vi "Snap.vi"(8 "error in (no error)":errorcluster, 11 "VisionUI in":refnum<class "VisionUI.lvclass">) -> (0 "error out":errorcluster, 3 "VisionUI out":refnum<class "VisionUI.lvclass">)   [LabVIEW 2021, in "VisionUI.lvlib" / "VisionUI.lvclass"]
uses:
  VisionUI.lvclass
  C:/Users/alan0/Desktop/WebSocket/Actors/Vision/Vision/Vision.lvclass
  VisionUI.lvclass/VisionUI.ctl
  Vision/Vision/Vision.lvclass
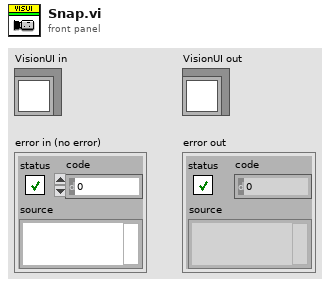
[diagram p1: front panel]
types:
  T1 = typedef "IMAQ Image.ctl" = refnum<image>
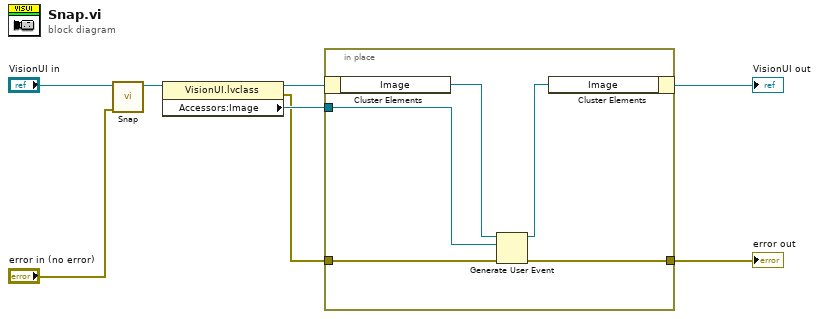
[diagram p0: block diagram]
diagram:
  n1 = call-parent "Snap.vi"("error in (no error)"="error in (no error)", "Vision in"="VisionUI in") -> ("Vision out"=w8:refnum<class "VisionUI.lvclass">)  [unwired: 8 in, 1 out]
  n2 = property class="VisionUI.lvclass"(reference=w8) -> (reference out=w5:refnum<class "VisionUI.lvclass">, error out=w2:errorcluster, "Accessors:Image"=w3:T1)  [unwired: 1 in]
  n3 = in-place {
    in-place-border: w3 -> [w11]
    in-place-border: w2 -> [w10]
    in-place-border: [w9] -> w1
    n4 = in-place-cluster #1(w5) -> ("Image"=w13:refnum<user-event>)
    n5 = Generate User Event(user event=w13, event data cluster=w11, error in=w10) -> (user event out=w12:refnum<user-event>, error out=w9:errorcluster)  [unwired: 1 in]
    n6 = in-place-cluster #1("Image"=w12) -> (→"VisionUI out":refnum<class "VisionUI.lvclass">)
  }
  "error out" <- w1
